vi "Save KML File.vi"(7 "KML File Path":path, 8 "error in (no error)":errorcluster, 9 "Altitude (m)":dbl, 10 "Longitude":dbl, 11 "Latitude":dbl) -> (0 "error out":errorcluster)   [LabVIEW 2013]
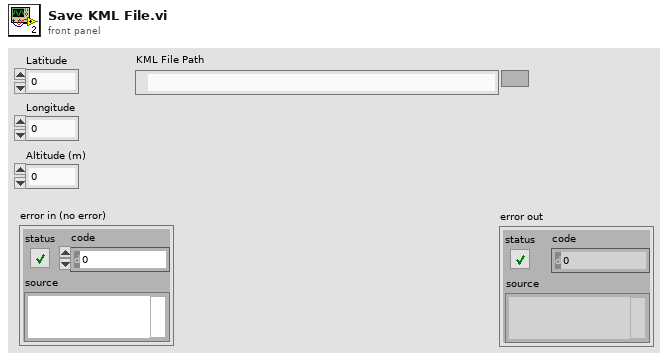
[diagram p1: front panel]
types:
  T1 = enum16{"open", "replace", "create", "open or create", "replace or create", "replace or create with confirmation"}
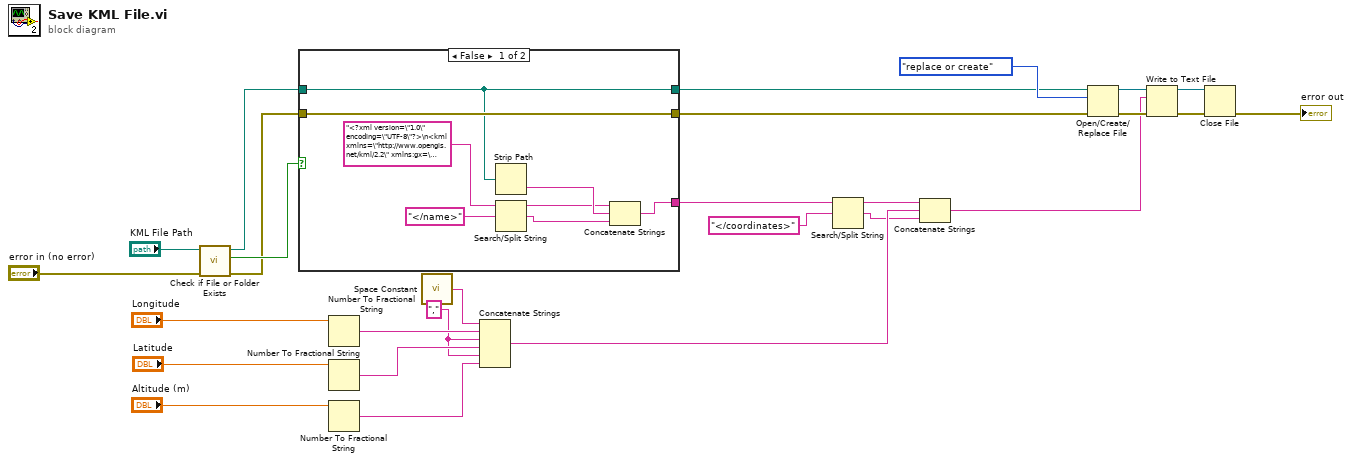
[diagram p0: block diagram]
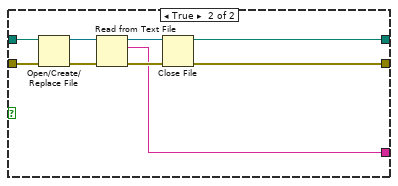
[diagram p2: hidden frame]
diagram:
  w21 = ","
  n1 = call <vilib>:"Check if File or Folder Exists.vi"("error in (no error)"="error in (no error)", "path"="KML File Path") -> ("error out"=w12:errorcluster, "file or folder exists?"=w14:bool, "dup path"=w13:path)  [unwired: 7 in]
  n2 = case shown="False" w14 {
    tunnel: [w28 w37] -> w1
    tunnel: [w35 w40] -> w9
    tunnel: w12 -> [w35 w39]
    tunnel: w13 -> [w29 w38]
    tunnel: [w29 w36] -> w8
    frame False {
      n3 = Strip Path(path=w29) -> (name=w33:string)  [unwired: 1 out]
      n4 = Search/Split String(string="<?xml version=\"1.0\" encoding=\"UTF-8\"?>\n<kml xmlns=\"http://www.opengis.net/kml/2.2\" xmlns:gx=\"http://www.google.com/kml/ext/2.2\" xmlns:kml=\"http://www.opengis.net/kml/2.2\" xmlns:atom=\"http://www.w3.org/2005/Atom\">\n<Document>\n\t<name></name>\n\t<StyleMap id=\"msn_ylw-pushpin\">\n\t\t<Pair>\n\t\t\t<key>normal</key>\n\t\t\t<styleUrl>#sn_ylw-pushpin</styleUrl>\n\t\t</Pair>\n\t\t<Pair>\n\t\t\t<key>highlight</key>\n\t\t\t<styleUrl>#sh_ylw-pushpin</styleUrl>\n\t\t</Pair>\n\t</StyleMap>\n\t<Style id=\"sh_ylw-pushpin\">\n\t\t<IconStyle>\n\t\t\t<scale>1.3</scale>\n\t\t\t<Icon>\n\t\t\t\t<href>http://maps.google.com/mapfiles/kml/pushpin/ylw-pushpin.png</href>\n\t\t\t</Icon>\n\t\t\t<hotSpot x=\"20\" y=\"2\" xunits=\"pixels\" yunits=\"pixels\"/>\n\t\t</IconStyle>\n\t\t<LineStyle>\n\t\t\t<color>ff00ffff</color>\n\t\t\t<width>3</width>\n\t\t</LineStyle>\n\t</Style>\n\t<Style id=\"sn_ylw-pushpin\">\n\t\t<IconStyle>\n\t\t\t<scale>1.1</scale>\n\t\t\t<Icon>\n\t\t\t\t<href>http://maps.google.com/mapfiles/kml/pushpin/ylw-pushpin.png</href>\n\t\t\t</Icon>\n\t\t\t<hotSpot x=\"20\" y=\"2\" xunits=\"pixels\" yunits=\"pixels\"/>\n\t\t</IconStyle>\n\t\t<LineStyle>\n\t\t\t<color>ff00ffff</color>\n\t\t\t<width>3</width>\n\t\t</LineStyle>\n\t</Style>\n\t<Placemark>\n\t\t<name>Balloon Path</name>\n\t\t<styleUrl>#msn_ylw-pushpin</styleUrl>\n\t\t<LineString>\n\t\t\t<tessellate>1</tessellate>\n\t\t\t<altitudeMode>absolute</altitudeMode>\n\t\t\t<coordinates>\n\t\t\t</coordinates>\n\t\t</LineString>\n\t</Placemark>\n</Document>\n</kml>\n", search string/char (-)="</name>") -> (substring before match=w32:string, match + rest of string=w34:string)  [unwired: 1 in, 1 out]
      n5 = Concatenate Strings(w32, w33, w34) -> (w28:string)
    }
    frame True {
      n6 = Open/Create/Replace File(file path (use dialog)=w38, error in=w39) -> (refnum out=w44:refnum<file>, error out=w43:errorcluster)  [unwired: 4 in, 1 out]
      n7 = Read from Text File(file (use dialog)=w44, error in=w43) -> (refnum out=w41:refnum<file>, text=w37:string, error out=w42:errorcluster)  [unwired: 2 in, 1 out]
      n8 = Close File(refnum=w41, error in=w42) -> (path=w36:path, error out=w40:errorcluster)
    }
  }
  n9 = Number To Fractional String(number="Longitude") -> (F-format string=w25:string)  [unwired: 3 in]
  n10 = Number To Fractional String(number="Latitude") -> (F-format string=w24:string)  [unwired: 3 in]
  n11 = Number To Fractional String(number="Altitude (m)") -> (F-format string=w23:string)  [unwired: 3 in]
  n12 = call <vilib>:"Space Constant.vi"() -> ("String"=w22:string)
  n13 = Concatenate Strings(w22, w25, w21, w24, w21, w23) -> (w19:string)
  n14 = Search/Split String(string=w1, search string/char (-)="</coordinates>") -> (substring before match=w20:string, match + rest of string=w18:string)  [unwired: 1 in, 1 out]
  n15 = Concatenate Strings(w20, w19, w18) -> (w5:string)
  n16 = Open/Create/Replace File(file path (use dialog)=w8, error in=w9, operation (0:open)=T1."replace or create") -> (refnum out=w6:refnum<file>, error out=w7:errorcluster)  [unwired: 3 in, 1 out]
  n17 = Write to Text File(file (use dialog)=w6, text=w5, error in=w7) -> (refnum out=w3:refnum<file>, error out=w4:errorcluster)  [unwired: 1 in, 1 out]
  n18 = Close File(refnum=w3, error in=w4) -> (error out=→"error out":errorcluster)  [unwired: 1 out]
